vi "Actor Core.vi"(8 "error in":errorcluster, 11 "UI Actor in":refnum<class "UI Actor.lvclass">) -> (0 "error out":errorcluster, 3 "Actor out":refnum<class "Actor.lvclass">)   [LabVIEW 2024, in "UI Actor.lvlib" / "UI Actor.lvclass"]
doc: "<p>(<strong>Filename</strong>: <span class=\"dnl\">Actor Framework.lvlib:Actor.lvclass:Actor Core.vi</span>)</p>\n<p>Receives messages to the actor, reacts to them, and initiates any error handling that may shut the actor down.</p>\n<p>Descendant classes may override this VI to append parallel tasks for the actor to complete while it handles messages. Overrides use the <a href=\"nihelplauncher://docs/csh?context=lvcore_glang_udclass\">Call Parent Class Method</a> node.</p>"
uses:
  UI Actor.lvclass
  <vilib>/ActorFramework/Actor/Actor.lvclass
  Controls/Device Info.ctl
  Controls/File Info.ctl
  Controls/Device Settings.ctl
  Controls/Supported Baudrates.ctl
  Core/Object Type.ctl
  Core/Data Type.ctl
  Core/Access SDO.ctl
  Core/Access PDO.ctl
  Core/Access SRDO.ctl
  <vilib>/Utility/miscctls.llb/LVRowAndColumnTypeDef.ctl
  UI Actor.lvclass/UI Actor.ctl
  UI Actor Messages/Populate Attributes Table Msg/Populate Attributes Table Msg.lvclass/Populate Attributes Table Msg.ctl
  <vilib>/ActorFramework/Message Enqueuer/Message Enqueuer.lvclass/Message Enqueuer.ctl
  UI Actor Messages/Populate Attribute Details Msg/Populate Attribute Details Msg.lvclass/Populate Attribute Details Msg.ctl
  UI Actor Messages/Read EDS File Msg/Read EDS File Msg.lvclass/Read EDS File Msg.ctl
  <vilib>/ActorFramework/Message Enqueuer/Enqueue.vi
  UI Actor Messages/Populate Attributes Table Msg/Populate Attributes Table Msg.lvclass
  UI Actor Messages/Populate Attribute Details Msg/Populate Attribute Details Msg.lvclass
  UI Actor Messages/Read EDS File Msg/Read EDS File Msg.lvclass
  <vilib>/ActorFramework/Stop Msg/Stop Msg.lvclass
  <vilib>/Utility/LVClass/Get LV Class Name.vi
  <resource>/AFDebug/Generate Trace for Message.vi
  <vilib>/ActorFramework/Message Priority Queue/Priority Enqueue.vi
  <vilib>/MGI/Panel Manager/Panel Actor/Panel Actor/Panel Actor.lvclass
  Core/EDS.lvlib
panel:
  in  "Filenames":i32(listbox)
  in  "Tab Control":T1(tab)
  out "auto":bool
  in  "Update Button":bool
  out "Concrete Node ID":string
  out "Device Settings":T2
  out "PDOs":T3
  out "File Info":T4={"FileVersion"=0, "FileRevision"=1, "EDSVersion"="", "Description"="", "CreationDate"="", "CreationTime"="", "CreatedBy"="", "ModificationDate"="", "ModificationTime"="", "ModifiedBy"=""}
  out "DeviceInfo":T5
  out "Baudrates":T6
  in  "DefaultValue":string
  in  "Actual Value":string
  in  "Access SRDO":T7
  in  "Access PDO":T8
  in  "Access SDO":T9
  in  "LowLimit":string
  in  "HighLimit":string
  in  "DataType":T10 items=["", "BOOLEAN", "INTEGER8", "INTEGER16", "INTEGER32", "UNSIGNED8", "UNSIGNED16", "UNSIGNED32", "REAL32", "VISIBLE_STRING", "OCTET_STRING", "UNICODE_STRING", "TIME_OF_DAY", "TIME_DIFFERENCE", "RESERVED1", "DOMAIN", "INTEGER24", "REAL64", "INTEGER40", "INTEGER48", "INTEGER56", "INTEGER64", "UNSIGNED24", "RESERVED2", "UNSIGNED40", "UNSIGNED48", "UNSIGNED56", "UNSIGNED64", "RESERVED3", "RESERVED4", "RESERVED5", "RESERVED6", "PDO_COMMUNICATION_PARAMETER", "PDO_MAPPING", "SDO_PARAMETER", "IDENTITY", "RESERVED7"]
  out "ObjectType":T11 items=["UNKNOWN"=255, "NULL"=0, "DOMAIN"=2, "DEFTYPE"=5, "DEFSTRUCT"=6, "VAR"=7, "ARRAY"=8, "RECORD"=9]
  out "Sub-Index":string
  out "Index":string
  out "Attribute Table":string[][](table)
  out "Device Profile Specific":string[][](table)
  out "Manufacturer Specific":string[][](table)
  in  "Communication Specific":string[][](table)
  in  "ParameterName":string
  in  "Description":string
  in  "Denotation":string
  out "Available Objects for PDO":string[][](table)
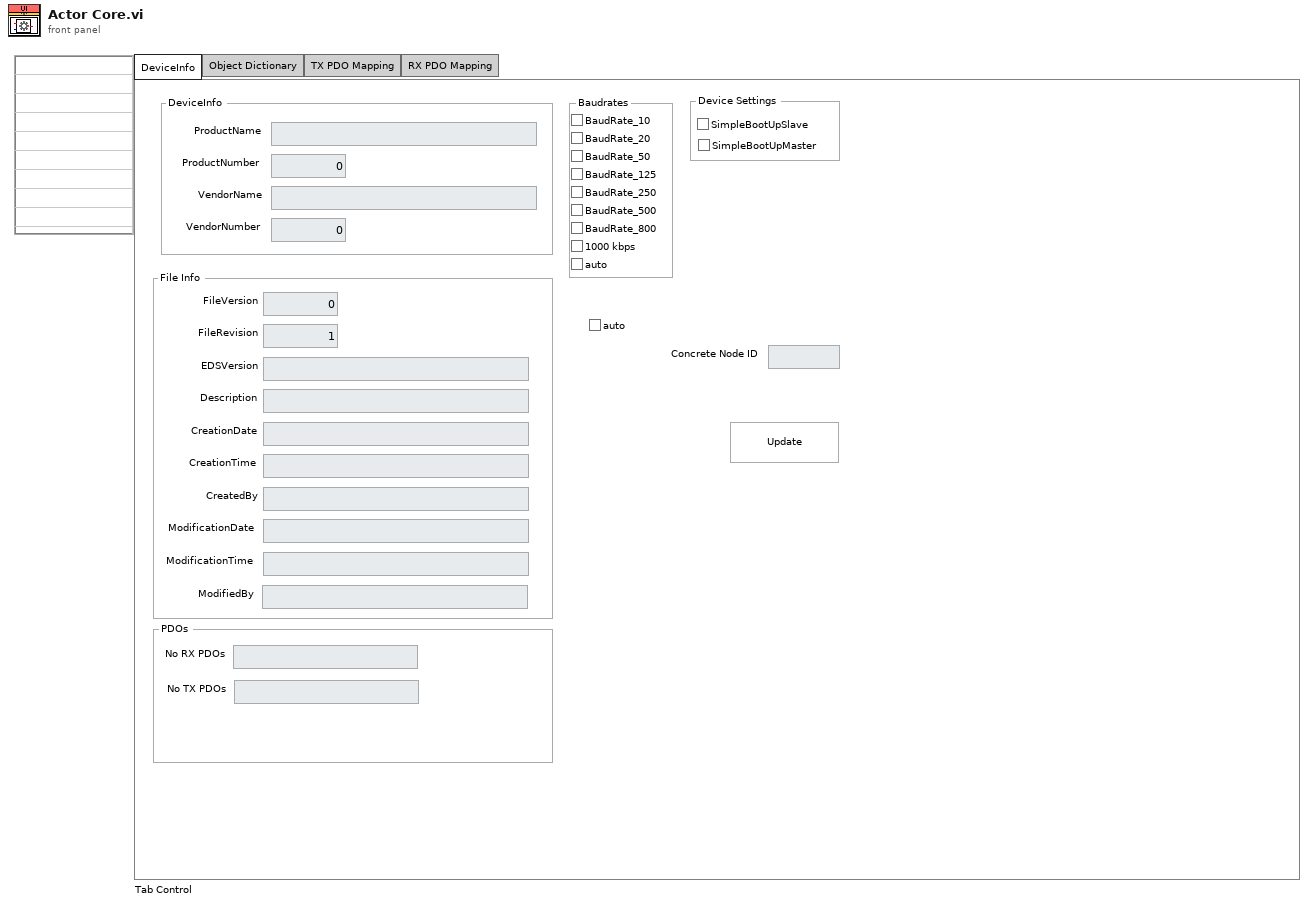
[diagram p1: front panel]
types:
  T1 = enum32{"DeviceInfo", "Object Dictionary", "TX PDO Mapping", "RX PDO Mapping"}
  T2 = typedef "Device Settings.ctl" = cluster{"SimpleBootUpSlave":bool, "SimpleBootUpMaster":bool}
  T3 = cluster{"No RX PDOs":string, "No TX PDOs":string}
  T4 = typedef "File Info.ctl" = cluster{"FileVersion":u8, "FileRevision":u8, "EDSVersion":string, "Description":string, "CreationDate":string, "CreationTime":string, "CreatedBy":string, "ModificationDate":string, "ModificationTime":string, "ModifiedBy":string}
  T5 = typedef "Device Info.ctl" = cluster{"ProductName":string, "ProductNumber":dbl, "VendorName":string, "VendorNumber":u32}
  T6 = typedef "Supported Baudrates.ctl" = cluster{"BaudRate_10":bool, "BaudRate_20":bool, "BaudRate_50":bool, "BaudRate_125":bool, "BaudRate_250":bool, "BaudRate_500":bool, "BaudRate_800":bool, "BaudRate_1000":bool, "BaudRate_auto":bool}
  T7 = typedef "EDS.lvlib/Access SRDO.ctl" = enum16{"no", "tx", "rx", "trx"}
  T8 = typedef "EDS.lvlib/Access PDO.ctl" = enum16{"no", "t", "r", "tr"}
  T9 = typedef "EDS.lvlib/Access SDO.ctl" = enum16{"no", "ro", "wo", "rw"}
  T10 = typedef "EDS.lvlib/Data Type.ctl" = u16
  T11 = typedef "EDS.lvlib/Object Type.ctl" = u8
  T12 = typedef "LVRowAndColumnTypeDef.ctl" = cluster{"Row":i32, "Column":i32}
  T13 = cluster{"DeviceInfo":refnum<user-event>, "Baudrates":refnum<user-event>, "File Info":refnum<user-event>, "Device Settings":refnum<user-event>, "Filenames":refnum<user-event>, "Communication Specific":refnum<user-event>, "Manufacturer Specific":refnum<user-event>, "Device Profile Specific":refnum<user-event>, "Attribute Table":refnum<user-event>, "Attribute Details":refnum<user-event>}
  T14 = cluster{"Pnl Actor":refnum<event-registration>, "Event Registration Refnum":refnum<event-registration>}
  T15 = enum8{"Enabled", "Disabled", "Disabled and Grayed Out"}
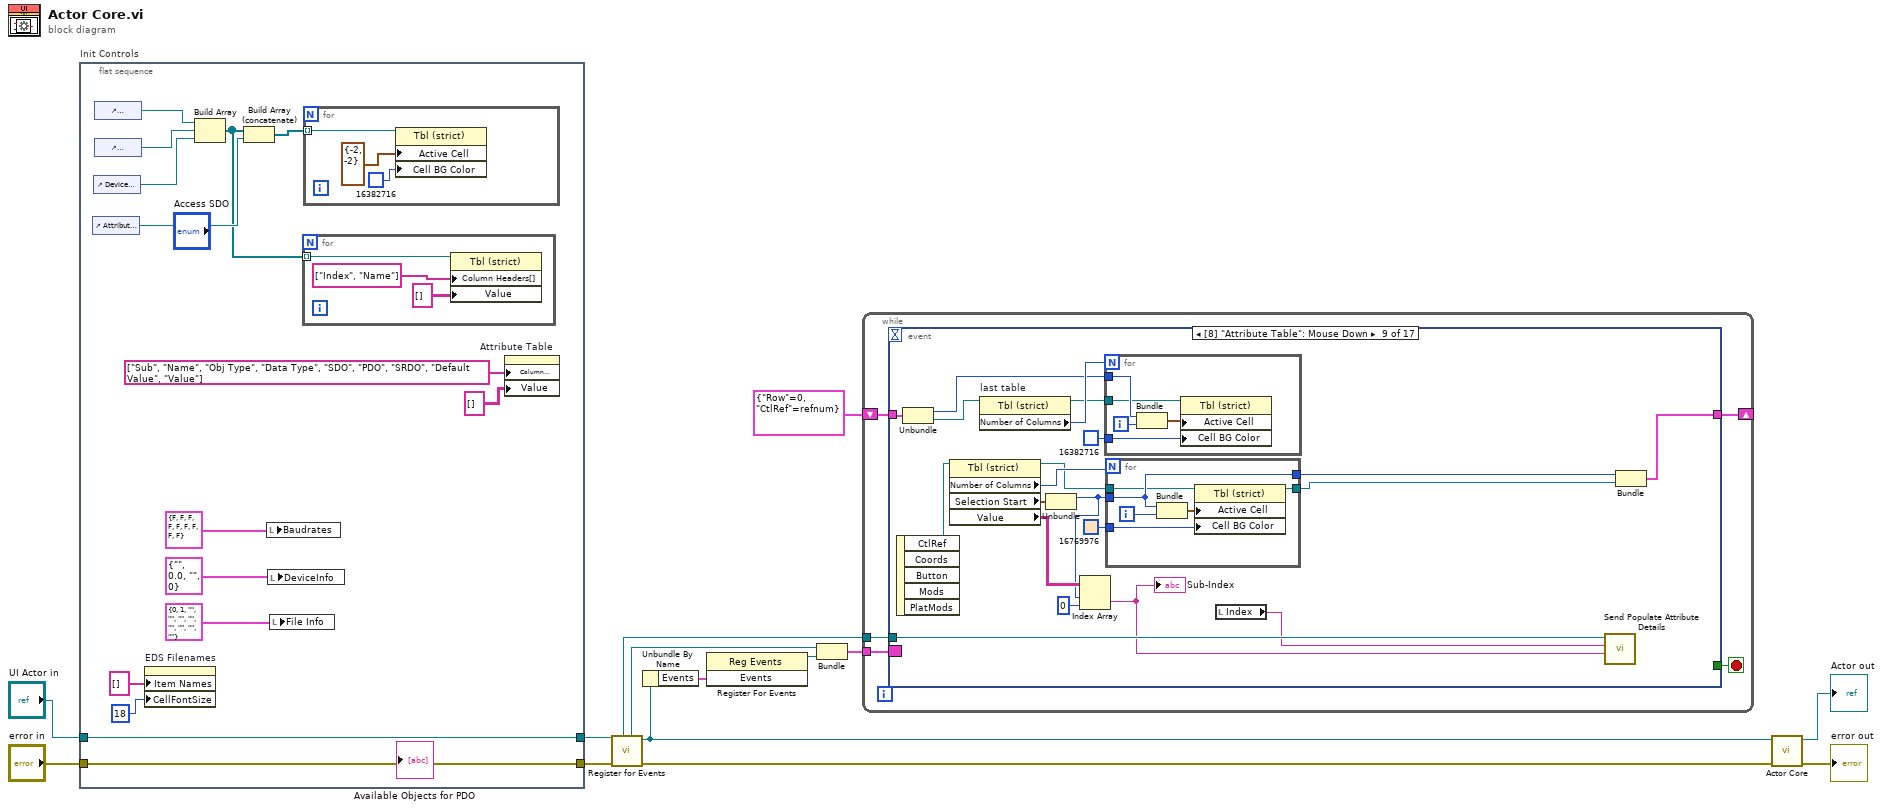
[diagram p0: block diagram]
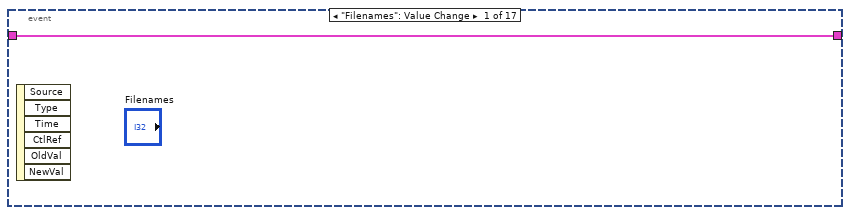
[diagram p2: hidden frame]
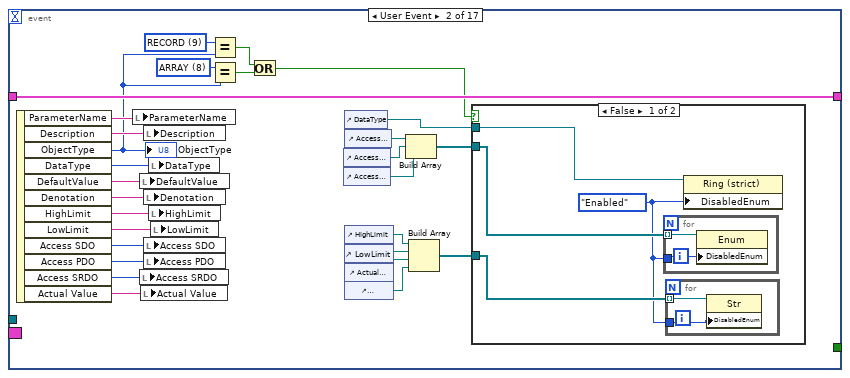
[diagram p3: hidden frame]
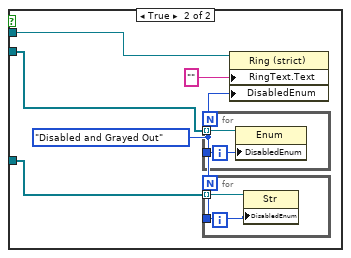
[diagram p4: hidden frame]
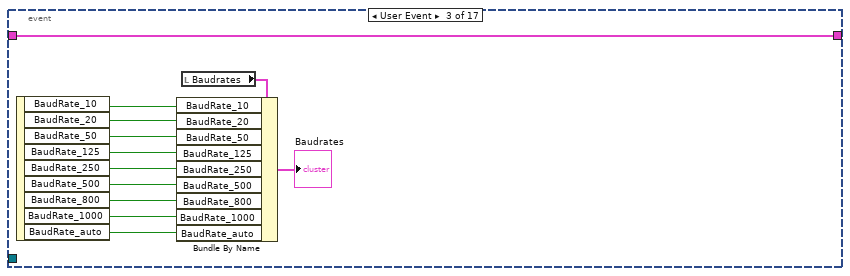
[diagram p5: hidden frame]
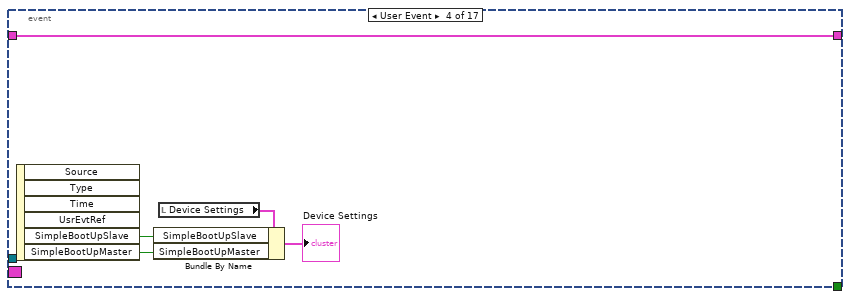
[diagram p6: hidden frame]
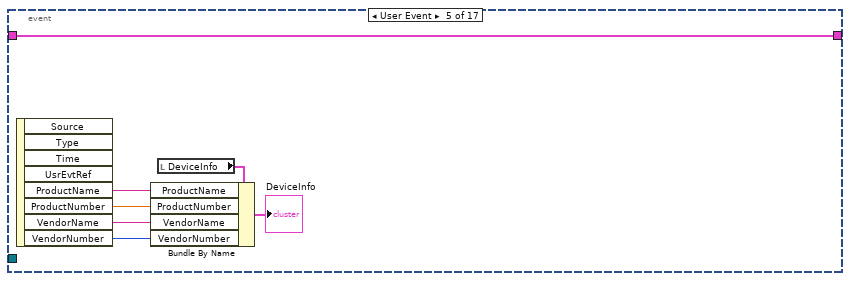
[diagram p7: hidden frame]
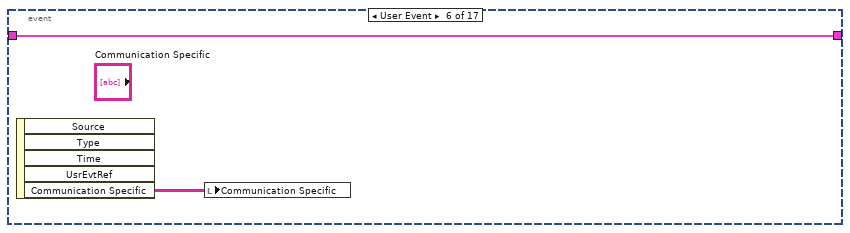
[diagram p8: hidden frame]
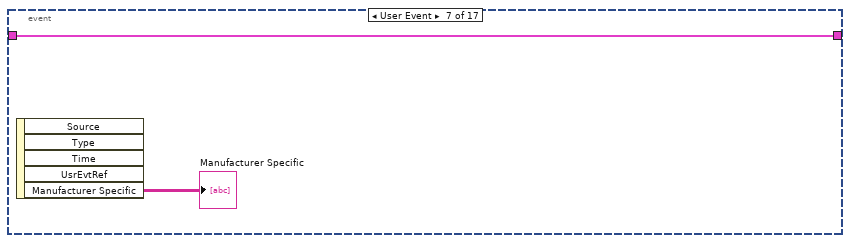
[diagram p9: hidden frame]
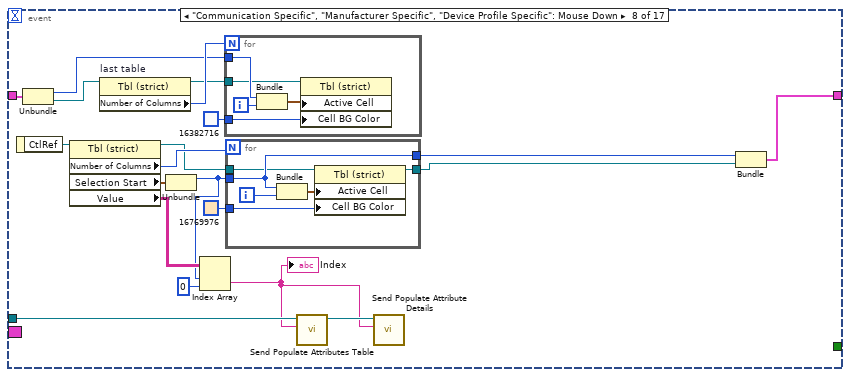
[diagram p10: hidden frame]
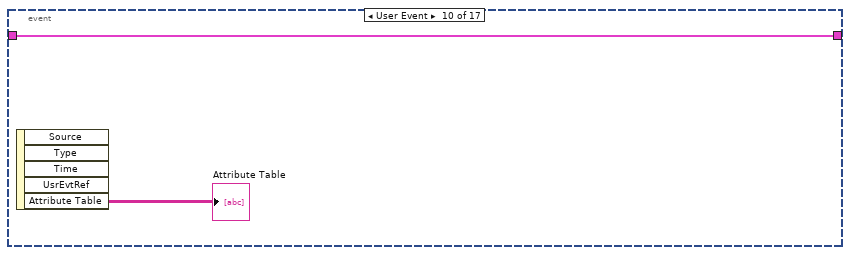
[diagram p11: hidden frame]
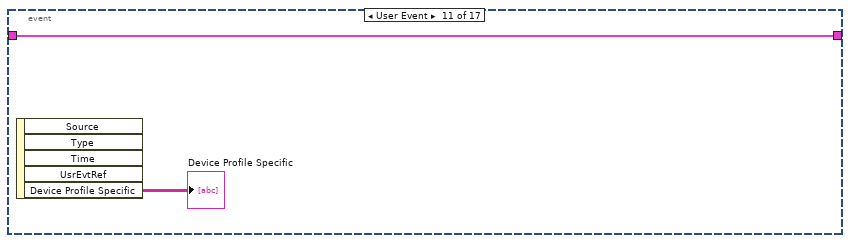
[diagram p12: hidden frame]
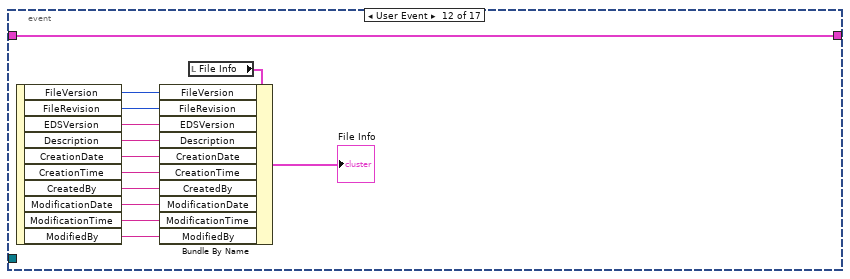
[diagram p13: hidden frame]
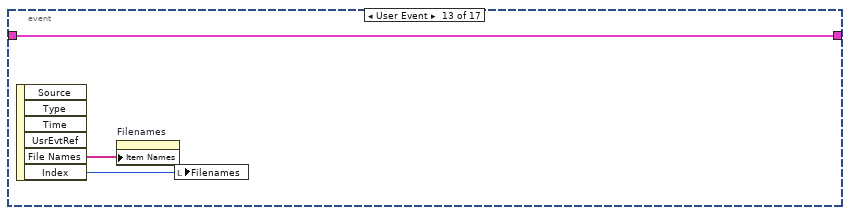
[diagram p14: hidden frame]
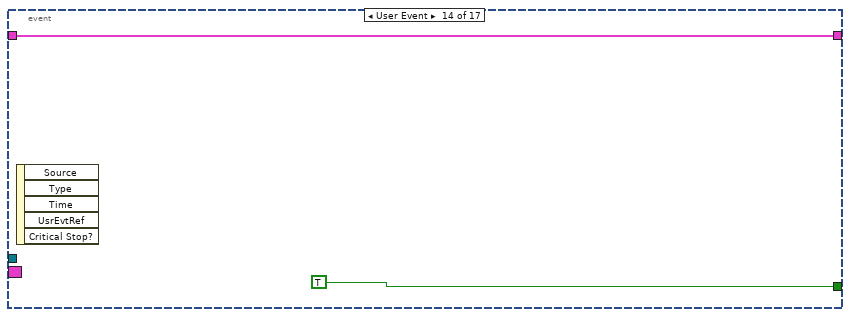
[diagram p15: hidden frame]
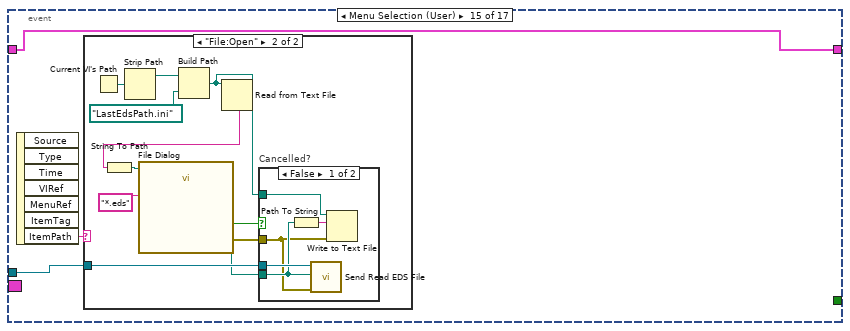
[diagram p16: hidden frame]
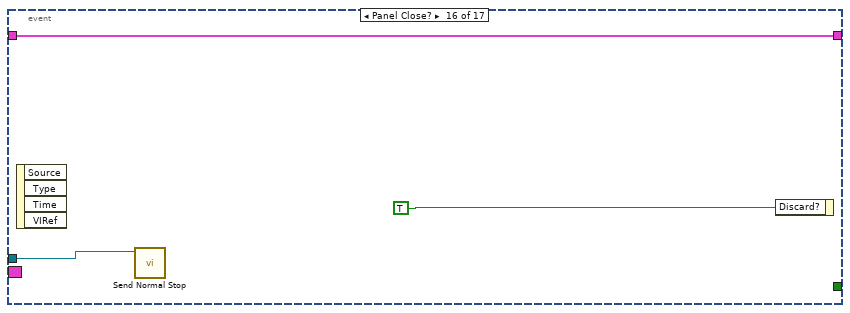
[diagram p19: hidden frame]
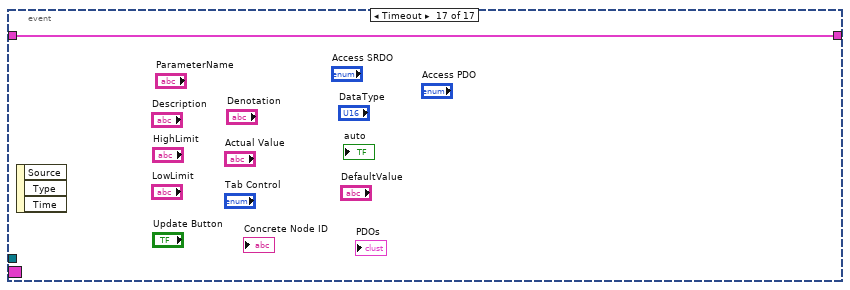
[diagram p20: hidden frame]
diagram:
  n1 = flat-sequence "Init Controls" {
    tunnel: "error in" -> [w15]
    tunnel: "UI Actor in" -> [w16]
    tunnel: [w15] -> w3
    tunnel: [w16] -> w2
    frame #0 {
      n2 = control-ref of="Attribute Table"() -> (w18:refnum<vi>)
      n3 = control-ref of="Device Profile Specific"() -> (w20:refnum<vi>)
      n4 = control-ref of="Communication Specific"() -> (w22:refnum<vi>)
      n5 = control-ref of="Manufacturer Specific"() -> (w21:refnum<vi>)
      n6 = property on="EDS Filenames" class="LstBox (strict)"("Item Names"=string[] [], "CellFontSize"=u32 18 ("Size:Height")) -> ()  [unwired: 2 in, 2 out]
      n7 = Build Array(w22, w21, w20) -> (w17:refnum<vi>[])
      n8 = Build Array (concatenate)(w17, w18) -> (w19:refnum<vi>[])
      n9 = local write "Baudrates"(T6 {"BaudRate_10"=FALSE, "BaudRate_20"=FALSE, "BaudRate_50"=FALSE, "BaudRate_125"=FALSE, "BaudRate_250"=FALSE, "BaudRate_500"=FALSE, "BaudRate_800"=FALSE, "BaudRate_1000"=FALSE, "BaudRate_auto"=FALSE} ("Baudrates")) -> ()
      n10 = local write "DeviceInfo"(T5 {"ProductName"="", "ProductNumber"=0.0, "VendorName"="", "VendorNumber"=0} ("DeviceInfo")) -> ()
      n11 = local write "File Info"(T4 {"FileVersion"=0, "FileRevision"=1, "EDSVersion"="", "Description"="", "CreationDate"="", "CreationTime"="", "CreatedBy"="", "ModificationDate"="", "ModificationTime"="", "ModifiedBy"=""} ("File Info")) -> ()
      n12 = for {
        tunnel: w17 -> [w30] mode=indexing
        n13 = property on="Property Node" class="Tbl (strict)"(reference=w30, "Column Headers[]"=string[] ["Index", "Name"] ("Compulsory Objects"), "Value"=string[][] [] ("Communication Specific")) -> ()  [unwired: 1 in, 2 out]
      }
      n14 = for {
        tunnel: w19 -> [w35] mode=indexing
        n15 = property class="Tbl (strict)"(reference=w35, "Active Cell"=T12 {"Row"=-2, "Column"=-2} ("Active Cell:Active Cell"), "Cell BG Color"=u32 16382716 ("Active Cell:Cell Background Color")) -> ()  [unwired: 1 in, 2 out]
      }
      n16 = property on="Attribute Table" class="Tbl (strict)"("Column Headers[]"=string[] ["Sub", "Name", "Obj Type", "Data Type", "SDO", "PDO", "SRDO", "Default Value", "Value"] ("Compulsory Objects"), "Value"=string[][] [] ("Communication Specific")) -> ()  [unwired: 2 in, 2 out]
    }
  }
  n17 = call <vilib>:"Register for Events.vi"("Error In"=w3, "Panel Actor in"=w2) -> ("Error Out"=w12:errorcluster, "Panel Actor out"=w8:refnum<class "UI Actor.lvclass">, "Pnl Actor"=w11:refnum<event-registration>, "Self Enqueuer"=w10:refnum<class "Message Enqueuer.lvclass">)  [unwired: 6 in]
  n18 = Unbundle By Name(w8) -> ("Events"=w7:T13)
  n19 = register-events(w7) -> (reference out=w6:refnum<event-registration>)  [unwired: 2 in, 1 out]
  n20 = Bundle("Pnl Actor"=w11, "Event Registration Refnum"=w6) -> (w9:T14)  [unwired: 1 in]
  n21 = while {
    tunnel: w9 -> [w39]
    tunnel: w10 -> [w38]
    shift-right: [w37] -> _
    shift-left: cluster{"Row":i32, "CtlRef":refnum<vi>} {"Row"=0, "CtlRef"=refnum} -> [w36]
    stop <- w40 stop-if-true
    n22 = event shown="[8] \"Attribute Table\": Mouse Down" {
      selector: w39 -> [_ _ _ _ _ _ _ _ _ _ _ _ _ _ _ _ _]
      dyn-events: _ -> [_ _ _ _ _ _ _ _ _ _ _ _ _ _ _ _ _]
      timeout: _ -> [_ _ _ _ _ _ _ _ _ _ _ _ _ _ _ _ _]
      tunnel: [_ _ _ _ _ _ _ _ _ _ _ _ _ TRUE _ _ _] -> w40
      tunnel: w38 -> [_ _ _ _ _ _ _ w119 w150 _ _ _ _ _ w200 w219 _]
      tunnel: [w41 w69 w87 w99 w104 w111 w113 w124 w155 w177 w179 w181 w194 w197 w199 w218 w221] -> w37
      tunnel: w36 -> [w41 w69 w87 w99 w104 w111 w113 w133 w164 w177 w179 w181 w194 w197 w199 w218 w221]
      event "Filenames": Value Change {
        n23 = event-data() -> ()  [unwired: 1 in, 6 out]
      }
      event User Event {
        w53 = T11 9 items=["NULL"=0, "DOMAIN"=2, "DEFTYPE"=5, "DEFSTRUCT"=6, "VAR"=7, "ARRAY"=8, "RECORD"=9] ("x")
        w54 = T11 8 items=["NULL"=0, "DOMAIN"=2, "DEFTYPE"=5, "DEFSTRUCT"=6, "VAR"=7, "ARRAY"=8, "RECORD"=9] ("x")
        n24 = event-data() -> ("ParameterName"=w68:string, "Description"=w67:string, "ObjectType"=w55:T11, "DataType"=w66:T10, "DefaultValue"=w65:string, "Denotation"=w64:string, "HighLimit"=w63:string, "LowLimit"=w62:string, "Access SDO"=w61:T9, "Access PDO"=w60:T8, "Access SRDO"=w59:T7, "Actual Value"=w58:string)  [unwired: 1 in]
        "ObjectType" <- w55
        n25 = local write "ParameterName"(w68) -> ()
        n26 = local write "DefaultValue"(w65) -> ()
        n27 = local write "Access SRDO"(w59) -> ()
        n28 = local write "Actual Value"(w58) -> ()
        n29 = local write "Description"(w67) -> ()
        n30 = local write "Denotation"(w64) -> ()
        n31 = local write "Access SDO"(w61) -> ()
        n32 = local write "Access PDO"(w60) -> ()
        n33 = local write "DataType"(w66) -> ()
        n34 = local write "HighLimit"(w63) -> ()
        n35 = local write "LowLimit"(w62) -> ()
        n36 = Equal?(x=w53, y=w55) -> (x = y?=w56:bool)
        n37 = Equal?(x=w54, y=w55) -> (x = y?=w57:bool)
        n38 = Or(x=w56, y=w57) -> (x .or. y?=w43:bool)
        n39 = control-ref of="Access PDO"() -> (w51:refnum<vi>)
        n40 = control-ref of="Access SRDO"() -> (w50:refnum<vi>)
        n41 = control-ref of="DataType"() -> (w42:refnum<vi>)
        n42 = control-ref of="Access SDO"() -> (w52:refnum<vi>)
        n43 = control-ref of="HighLimit"() -> (w45:refnum<vi>)
        n44 = control-ref of="LowLimit"() -> (w46:refnum<vi>)
        n45 = control-ref of="Actual Value"() -> (w47:refnum<vi>)
        n46 = control-ref of="DefaultValue"() -> (w48:refnum<vi>)
        n47 = Build Array(w52, w51, w50) -> (w49:refnum<vi>[])
        n48 = Build Array(w45, w46, w47, w48) -> (w44:refnum<vi>[])
        n49 = case shown="False" w43 {
          tunnel: w49 -> [w72 w82]
          tunnel: w44 -> [w73 w81]
          tunnel: w42 -> [w71 w80]
          frame False {
            w70 = T15."Enabled" ("Disabled")
            n50 = for {
              tunnel: w72 -> [w77] mode=indexing
              tunnel: w70 -> [w76]
              n51 = property on="Property Node" class="Enum"(reference=w77, "DisabledEnum"=w76) -> ()  [unwired: 1 in, 2 out]
            }
            n52 = for {
              tunnel: w73 -> [w75] mode=indexing
              tunnel: w70 -> [w74]
              n53 = property on="Property Node" class="Str"(reference=w75, "DisabledEnum"=w74) -> ()  [unwired: 1 in, 2 out]
            }
            n54 = property on="Property Node" class="Ring (strict)"(reference=w71, "DisabledEnum"=w70) -> ()  [unwired: 1 in, 2 out]
          }
          frame True {
            w78 = T15."Disabled and Grayed Out" ("Disabled")
            n55 = for {
              tunnel: w82 -> [w86] mode=indexing
              tunnel: w78 -> [w85]
              n56 = property on="Property Node" class="Enum"(reference=w86, "DisabledEnum"=w85) -> ()  [unwired: 1 in, 2 out]
            }
            n57 = for {
              tunnel: w81 -> [w84] mode=indexing
              tunnel: w78 -> [w83]
              n58 = property on="Property Node" class="Str"(reference=w84, "DisabledEnum"=w83) -> ()  [unwired: 1 in, 2 out]
            }
            n59 = property on="Property Node" class="Ring (strict)"(reference=w80, "RingText.Text"="" ("Ring Text.Text"), "DisabledEnum"=w78) -> ()  [unwired: 1 in, 2 out]
          }
        }
      }
      event User Event {
        n60 = event-data() -> ("BaudRate_10"=w97:bool, "BaudRate_20"=w96:bool, "BaudRate_50"=w95:bool, "BaudRate_125"=w94:bool, "BaudRate_250"=w93:bool, "BaudRate_500"=w92:bool, "BaudRate_800"=w91:bool, "BaudRate_1000"=w90:bool, "BaudRate_auto"=w88:bool)  [unwired: 1 in]
        n61 = local read "Baudrates"() -> (w98:T6)
        n62 = Bundle By Name(cluster=w98, "BaudRate_10"=w97, "BaudRate_20"=w96, "BaudRate_50"=w95, "BaudRate_125"=w94, "BaudRate_250"=w93, "BaudRate_500"=w92, "BaudRate_800"=w91, "BaudRate_1000"=w90, "BaudRate_auto"=w88) -> (→"Baudrates":T6)
      }
      event User Event {
        n63 = event-data() -> ("SimpleBootUpSlave"=w102:bool, "SimpleBootUpMaster"=w101:bool)  [unwired: 1 in, 4 out]
        n64 = local read "Device Settings"() -> (w103:T2)
        n65 = Bundle By Name(cluster=w103, "SimpleBootUpSlave"=w102, "SimpleBootUpMaster"=w101) -> (→"Device Settings":T2)
      }
      event User Event {
        n66 = event-data() -> ("ProductName"=w109:string, "ProductNumber"=w108:dbl, "VendorName"=w107:string, "VendorNumber"=w106:u32)  [unwired: 1 in, 4 out]
        n67 = local read "DeviceInfo"() -> (w110:T5)
        n68 = Bundle By Name(cluster=w110, "ProductName"=w109, "ProductNumber"=w108, "VendorName"=w107, "VendorNumber"=w106) -> (→"DeviceInfo":T5)
      }
      event User Event {
        n69 = event-data() -> ("Communication Specific"=w112:string[][])  [unwired: 1 in, 4 out]
        n70 = local write "Communication Specific"(w112) -> ()
      }
      event User Event {
        n71 = event-data() -> ("Manufacturer Specific"=→"Manufacturer Specific":string[][])  [unwired: 1 in, 4 out]
      }
      event "Communication Specific", "Manufacturer Specific", "Device Profile Specific": Mouse Down {
        n72 = event-data() -> ("CtlRef"=w121:refnum<vi>)  [unwired: 1 in]
        n73 = Unbundle(w133) -> ("Row"=w125:i32, "CtlRef"=w126:refnum<vi>)
        n74 = property class="Tbl (strict)"(reference=w121) -> (reference out=w129:refnum<vi>, "Number of Columns"=w132:u32, "Selection Start"=w134:T12, "Value"=w120:string[][])  [unwired: 1 in, 1 out]
        n75 = property on="last table" class="Tbl (strict)"(reference=w126) -> (reference out=w122:refnum<vi>, "Number of Columns"=w127:u32)  [unwired: 1 in, 1 out]
        n76 = Unbundle(w134) -> ("Row"=w117:i32)  [unwired: 1 out]
        n77 = Index Array(array=w120, index (row)=w117, index (col)=0) -> (element=w115:string)
        "Index" <- w115
        n78 = for {
          N: w127 -> [_]
          tunnel: u32 16382716 ("Active Cell:Cell Background Color") -> [w145]
          tunnel: w125 -> [w142]
          tunnel: w122 -> [w141]
          i -> [w144]
          n79 = Bundle("Row"=w142, w144) -> (w143:cluster{"Row":i32, i32})  [unwired: 1 in]
          n80 = property class="Tbl (strict)"(reference=w141, "Active Cell"=w143, "Cell BG Color"=w145) -> ()  [unwired: 1 in, 2 out]
        }
        n81 = for {
          N: w132 -> [_]
          tunnel: w117 -> [w139]
          tunnel: u32 16769976 -> [w138]
          tunnel: [w139] -> w130
          tunnel: w129 -> [w136]
          tunnel: [w135] -> w123
          i -> [w140]
          n82 = Bundle("Row"=w139, w140) -> (w137:cluster{"Row":i32, i32})  [unwired: 1 in]
          n83 = property class="Tbl (strict)"(reference=w136, "Active Cell"=w137, "Cell BG Color"=w138) -> (reference out=w135:refnum<vi>)  [unwired: 1 in, 1 out]
        }
        n84 = call "Send Populate Attributes Table.vi"("Index"=w115, "Message Enqueuer"=w119) -> ("Message Enqueuer out"=w116:refnum<class "Message Enqueuer.lvclass">)  [unwired: 8 in, 1 out]
        n85 = call "Send Populate Attribute Details.vi"("Index"=w115, "Message Enqueuer"=w116) -> ()  [unwired: 8 in, 2 out]
        n86 = Bundle("Row"=w130, "CtlRef"=w123) -> (w124:cluster{"Row":i32, "CtlRef":refnum<vi>})  [unwired: 1 in]
      }
      event "Attribute Table": Mouse Down {
        n87 = event-data() -> ("CtlRef"=w152:refnum<vi>)  [unwired: 1 in, 4 out]
        n88 = Unbundle(w164) -> ("Row"=w156:i32, "CtlRef"=w157:refnum<vi>)
        n89 = property class="Tbl (strict)"(reference=w152) -> (reference out=w160:refnum<vi>, "Number of Columns"=w163:u32, "Selection Start"=w165:T12, "Value"=w151:string[][])  [unwired: 1 in, 1 out]
        n90 = property on="last table" class="Tbl (strict)"(reference=w157) -> (reference out=w153:refnum<vi>, "Number of Columns"=w158:u32)  [unwired: 1 in, 1 out]
        n91 = Unbundle(w165) -> ("Row"=w148:i32)  [unwired: 1 out]
        n92 = Index Array(array=w151, index (row)=w148, index (col)=0) -> (element=w146:string)
        "Sub-Index" <- w146
        n93 = for {
          N: w158 -> [_]
          tunnel: u32 16382716 ("Active Cell:Cell Background Color") -> [w176]
          tunnel: w156 -> [w173]
          tunnel: w153 -> [w172]
          i -> [w175]
          n94 = Bundle("Row"=w173, w175) -> (w174:cluster{"Row":i32, i32})  [unwired: 1 in]
          n95 = property class="Tbl (strict)"(reference=w172, "Active Cell"=w174, "Cell BG Color"=w176) -> ()  [unwired: 1 in, 2 out]
        }
        n96 = for {
          N: w163 -> [_]
          tunnel: w148 -> [w170]
          tunnel: u32 16769976 -> [w169]
          tunnel: [w170] -> w161
          tunnel: w160 -> [w167]
          tunnel: [w166] -> w154
          i -> [w171]
          n97 = Bundle("Row"=w170, w171) -> (w168:cluster{"Row":i32, i32})  [unwired: 1 in]
          n98 = property class="Tbl (strict)"(reference=w167, "Active Cell"=w168, "Cell BG Color"=w169) -> (reference out=w166:refnum<vi>)  [unwired: 1 in, 1 out]
        }
        n99 = local read "Index"() -> (w147:string)
        n100 = call "Send Populate Attribute Details.vi"("Sub-Index"=w146, "Index"=w147, "Message Enqueuer"=w150) -> ()  [unwired: 7 in, 2 out]
        n101 = Bundle("Row"=w161, "CtlRef"=w154) -> (w155:cluster{"Row":i32, "CtlRef":refnum<vi>})  [unwired: 1 in]
      }
      event User Event {
        n102 = event-data() -> ("Attribute Table"=→"Attribute Table":string[][])  [unwired: 1 in, 4 out]
      }
      event User Event {
        n103 = event-data() -> ("Device Profile Specific"=→"Device Profile Specific":string[][])  [unwired: 1 in, 4 out]
      }
      event User Event {
        n104 = event-data() -> ("FileVersion"=w183:u8, "FileRevision"=w184:u8, "EDSVersion"=w185:string, "Description"=w186:string, "CreationDate"=w187:string, "CreationTime"=w188:string, "CreatedBy"=w189:string, "ModificationDate"=w190:string, "ModificationTime"=w191:string, "ModifiedBy"=w192:string)  [unwired: 1 in]
        n105 = local read "File Info"() -> (w193:T4)
        n106 = Bundle By Name(cluster=w193, "FileVersion"=w183, "FileRevision"=w184, "EDSVersion"=w185, "Description"=w186, "CreationDate"=w187, "CreationTime"=w188, "CreatedBy"=w189, "ModificationDate"=w190, "ModificationTime"=w191, "ModifiedBy"=w192) -> (→"File Info":T4)
      }
      event User Event {
        n107 = event-data() -> ("File Names"=w196:string[], "Index"=w195:i32)  [unwired: 1 in, 4 out]
        n108 = property on="Filenames" class="LstBox (strict)"("Item Names"=w196) -> ()  [unwired: 2 in, 2 out]
        n109 = local write "Filenames"(w195) -> ()
      }
      event User Event {
        n110 = event-data() -> ()  [unwired: 1 in, 5 out]
      }
      event Menu Selection (User) {
        n111 = event-data() -> ("ItemPath"=w201:string)  [unwired: 1 in, 6 out]
        n112 = case shown="\"File:Open\"" w201 {
          tunnel: w200 -> [_ w210]
          frame "False", Default {
          }
          frame "File:Open" {
            n113 = Current VI's Path() -> (path=w208:path)
            n114 = Strip Path(path=w208) -> (stripped path=w204:path)  [unwired: 1 out]
            n115 = Build Path(base path=w204, name or relative path=path "LastEdsPath.ini") -> (appended path=w202:path)
            n116 = Read from Text File(file (use dialog)=w202) -> (text=w207:string)  [unwired: 3 in, 3 out]
            n117 = String To Path(string=w207) -> (path=w206:path)
            n118 = call "File Dialog"("start path"=w206, "pattern (all files)"="*.eds") -> ("selected path"=w205:path, "cancelled"=w209:bool, "error out"=w212:errorcluster)  [unwired: 10 in, 1 out]
            n119 = case "Cancelled?" shown="False" w209 {
              tunnel: w212 -> [w213 _]
              tunnel: w210 -> [w217 _]
              tunnel: w205 -> [w214 _]
              tunnel: w202 -> [w215 _]
              frame False {
                n120 = Path To String(path=w214) -> (string=w216:string)
                n121 = call "Send Read EDS File.vi"("error in (no error)"=w213, "EDS File Path"=w214, "Message Enqueuer"=w217) -> ()  [unwired: 7 in, 2 out]
                n122 = Write to Text File(file (use dialog)=w215, text=w216, error in=w213) -> ()  [unwired: 1 in, 3 out]
              }
              frame True {
              }
            }
          }
        }
      }
      event Panel Close? {
        n123 = event-data() -> ()  [unwired: 1 in, 4 out]
        n124 = call <vilib>:"Send Normal Stop.vi"("Message Enqueuer"=w219) -> ()  [unwired: 10 in, 1 out]
        n125 = event-data("Discard?"=TRUE) -> ()  [unwired: 1 in, 1 out]
      }
      event Timeout {
        n126 = event-data() -> ()  [unwired: 1 in, 3 out]
      }
    }
  }
  n127 = call-parent "Actor Core.vi"("error in"=w12, "Panel Actor in"=w8) -> ("error out"=→"error out":errorcluster, "Actor out"=→"Actor out":refnum<class "Actor.lvclass">)  [unwired: 8 in]
